vi "LCD_I2C.vi"(8 "error in (no error)":errorcluster, 10 "Cluster LCD":T1={"Direccion"=4, "Columna"=0, "Fila"=0, "Texto"=""} {"Fila" format="%x"; "Columna" format="%x"; "Direccion" min=4 max=40 format="%x"}, 11 "VISA resource name":refnum<visa-resource-name>) -> (0 "error out":errorcluster, 2 "read buffer":string, 3 "VISA resource name out":refnum<visa-resource-name>)   [LabVIEW 2025]
panel:
  # "NOTA: NO USAR con el SHIELD GALIOT la parte de I2C se pierde"
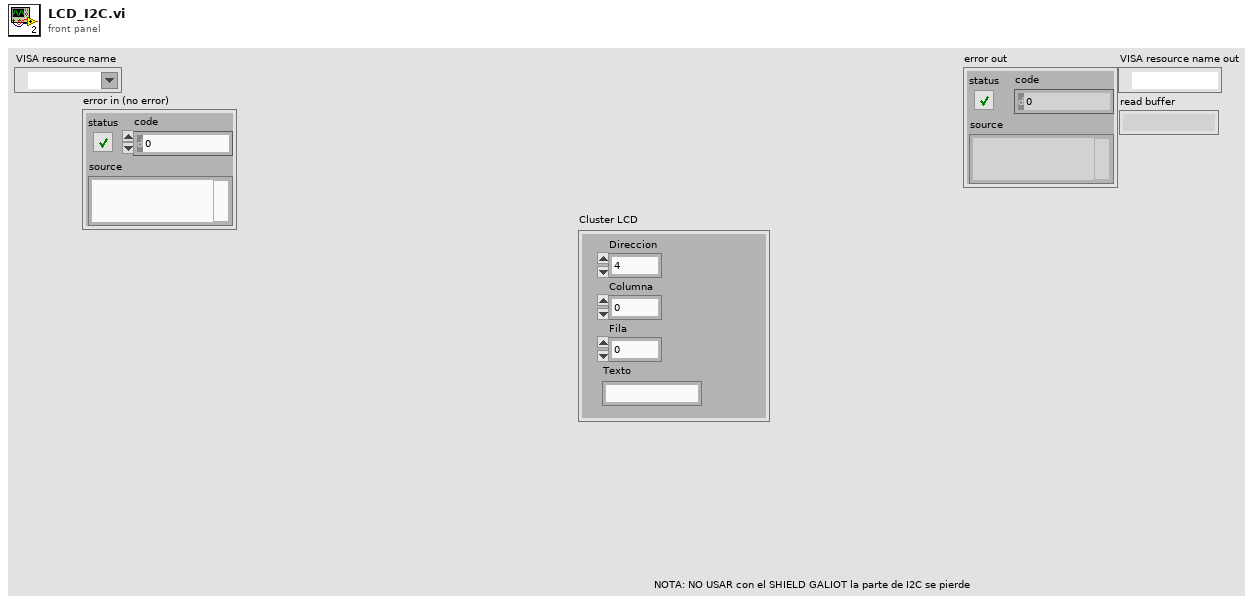
[diagram p1: front panel]
types:
  T1 = cluster{"Direccion":u8, "Columna":u8, "Fila":u8, "Texto":string}
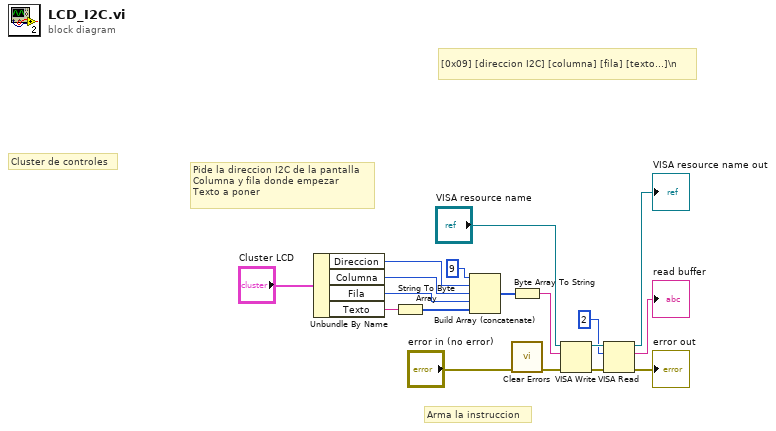
[diagram p0: block diagram]
diagram:
  # "Arma la instruccion"
  # "Pide la direccion I2C de la pantalla\nColumna y fila donde empezar\nTexto a poner"
  # "Cluster de controles"
  # "[0x09] [direccion I2C] [columna] [fila] [texto...]\\n"
  n1 = Unbundle By Name("Cluster LCD") -> ("Direccion"=w4:u8, "Columna"=w3:u8, "Fila"=w2:u8, "Texto"=w1:string)
  n2 = String To Byte Array(string=w1) -> (unsigned byte array=w6:u8[])
  n3 = Build Array (concatenate)(u8 9, w4, w3, w2, w6) -> (w16:u8[])
  n4 = Byte Array To String(unsigned byte array=w16) -> (string=w18:string)
  n5 = call <vilib>:"Clear Errors.vi"("error in (no error)"="error in (no error)") -> ("error out"=w14:errorcluster)  [unwired: 5 in, 1 out]
  n6 = VISA Write(VISA resource name="VISA resource name", write buffer=w18, error in (no error)=w14) -> (VISA resource name out=w9:refnum<visa-resource-name>, error out=w12:errorcluster)  [unwired: 1 out]
  n7 = VISA Read(VISA resource name=w9, byte count=u32 2, error in (no error)=w12) -> (VISA resource name out=→"VISA resource name out":refnum<visa-resource-name>, read buffer=→"read buffer":string, error out=→"error out":errorcluster)  [unwired: 1 out]
